vi "CheckLabVIEWMode.vi"(11 "Templates In":refnum<class "MetaDataObj.lvclass">[](array[class])) -> (3 "Templates Out":refnum<class "MetaDataObj.lvclass">[](array[class]))   [LabVIEW 2016, in "NI_NPW_Loading Project Info.lvlib"]
uses:
  <resource>/dialog/NewProjectWizard/Loading Project Info/NI_NPW_Loading Project Info.lvlib
  <resource>/dialog/NewProjectWizard/MetaDataObj/MetaDataObj.lvclass
  <resource>/dialog/NewProjectWizard/MetaDataObj/Accessors/Read Modes.vi
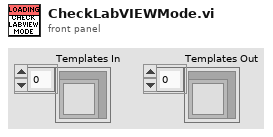
[diagram p1: front panel]
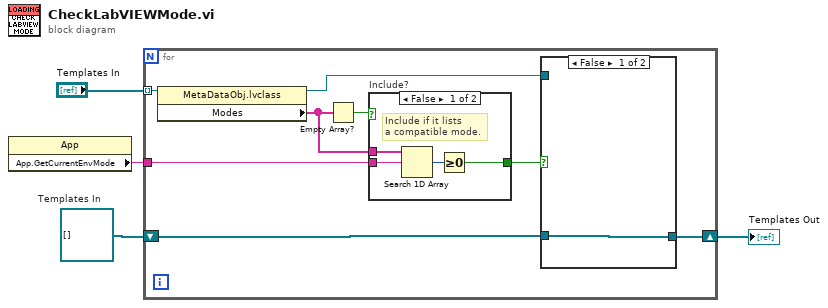
[diagram p0: block diagram]
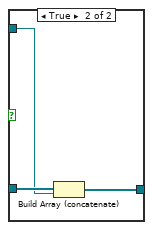
[diagram p2: hidden frame]
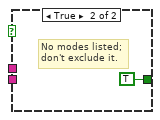
[diagram p3: hidden frame]
diagram:
  w4 = refnum<class "MetaDataObj.lvclass">[] []  # Templates In
  n1 = property class="App"() -> ("App.GetCurrentEnvMode"=w2:string)  [unwired: 2 in, 2 out]
  n2 = for {
    shift-right: [w7] -> w1
    shift-left: w4 -> [w8]
    tunnel: "Templates In" -> [w12] mode=indexing
    tunnel: w2 -> [w11]
    n3 = property class="MetaDataObj.lvclass"(reference=w12) -> (reference out=w10:refnum<class "MetaDataObj.lvclass">, "Modes"=w6:string[])  [unwired: 1 in, 1 out]
    n4 = Empty Array?(array=w6) -> (empty?=w5:bool)
    n5 = case "Include?" shown="False" w5 {
      tunnel: w6 -> [w20 _]
      tunnel: w11 -> [w19 _]
      tunnel: [w17 TRUE] -> w9
      frame False {
        # "Include if it lists\na compatible mode."
        n6 = Search 1D Array(1D array=w20, element=w19) -> (index of element=w18:i32)  [unwired: 1 in]
        n7 = Greater Or Equal To 0?(x=w18) -> (x >= 0?=w17:bool)
      }
      frame True {
        # "No modes listed;\ndon't exclude it."
      }
    }
    n8 = case shown="False" w9 {
      tunnel: w10 -> [_ w15]
      tunnel: w8 -> [w13 w16]
      tunnel: [w13 w14] -> w7
      frame False {
      }
      frame True {
        n9 = Build Array (concatenate)(w16, w15) -> (w14:refnum<class "MetaDataObj.lvclass">[])
      }
    }
  }
  "Templates Out" <- w1
